vi "myRIO_BRig_RT__Case_Exp_State_initTrial_dispense.vi"(10 "input_state":T1, 11 "input_dataMTrig":u16[](array[numeric])) -> (0 "output_dispense__R":bool, 1 "output_dispense__L":bool, 2 "output_state":T1, 3 "output_dataMTrig":u16[](array[numeric]))   [LabVIEW 2014]
uses:
  myRIO_Gil_RT_v1__states.vi
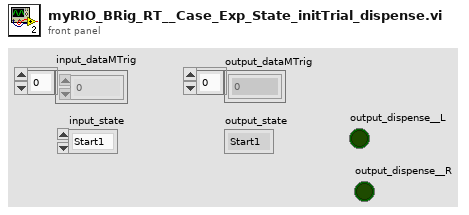
[diagram p1: front panel]
types:
  T1 = typedef "myRIO_Gil_RT_v1__states.vi" = enum16{"Start1", "Start2", "Start3", "initBlock", "initTrial", "initTrial_dispense_pre", "initTrial_dispense", "ENL1_pre", "ENL1", "ENL1Penalty_pre", "ENL1Penalty", "ENL2_pre", "ENL2", "ENL2Penalty_pre", "ENL2Penalty", "Cue1_pre", "Cue1", "Cue1Penalty_pre", "Cue1Penalty", "Cue2_pre", "Cue2", "Cue2Penalty_pre", "Cue2Penalty", "Selection_pre", "Selection", "SelectReward_pre", "SelectReward", "SelectRewardPost_pre", "SelectRewardPost", "SelectWrong_pre", "SelectWrong", "SelectTimeout_pre", "SelectTimeout", "SelectTimeout_post", "endTrial1", "endTrial2", "transferCheck", "transferPrepare", "transferCleanUp", "endBlock", "endExp"}
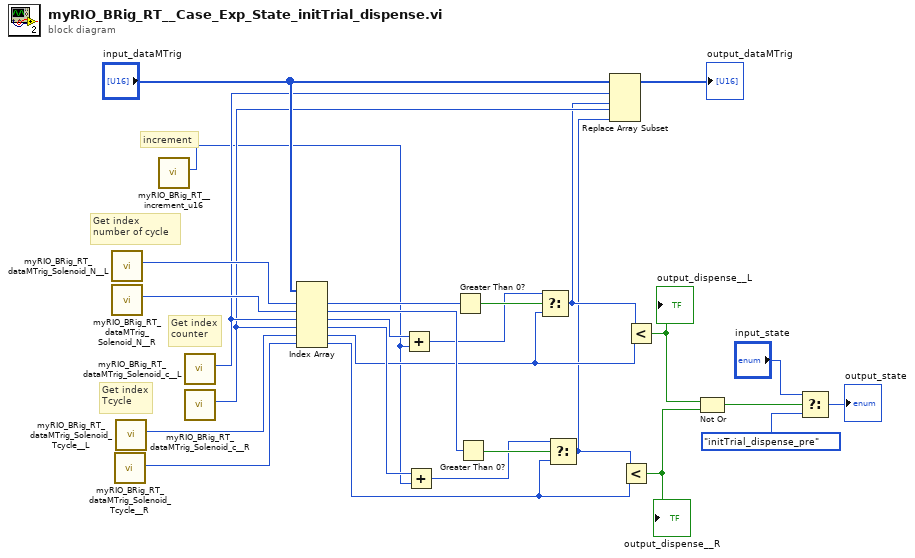
[diagram p0: block diagram]
diagram:
  # "increment"
  # "Get index\nTcycle"
  # "Get index\nnumber of cycle"
  # "Get index\ncounter"
  n1 = call "myRIO_BRig_RT_dataMTrig_Solenoid_N__L.vi"() -> ("output_Solenoid_N__L"=w27:i32)  [unwired: 11 in]
  n2 = call "myRIO_BRig_RT_dataMTrig_Solenoid_N__R.vi"() -> ("output_Solenoid_N__R"=w26:i32)  [unwired: 11 in]
  n3 = call "myRIO_BRig_RT_dataMTrig_Solenoid_Tcycle__R.vi"() -> ("output_Solenoid_Tcycle__R"=w24:i32)  [unwired: 11 in]
  n4 = call "myRIO_BRig_RT_dataMTrig_Solenoid_Tcycle__L.vi"() -> ("output_Solenoid_Tcycle__L"=w25:i32)  [unwired: 11 in]
  n5 = call "myRIO_BRig_RT__increment_u16.vi"() -> ("output_increment__u16"=w1:u16)  [unwired: 11 in]
  n6 = call "myRIO_BRig_RT_dataMTrig_Solenoid_c__L.vi"() -> ("output_Solenoid_c__L"=w11:i32)  [unwired: 11 in]
  n7 = call "myRIO_BRig_RT_dataMTrig_Solenoid_c__R.vi"() -> ("output_Solenoid_c__R"=w10:i32)  [unwired: 11 in]
  n8 = Index Array(array="input_dataMTrig", index #1=w27, index #2=w26, index #3=w11, index #4=w10, index #5=w25, index #6=w24) -> (element #1=w23:u16, element #2=w22:u16, element #3=w21:u16, element #4=w20:u16, element #5=w15:u16, element #6=w14:u16)
  n9 = Add(x=w21, y=w1) -> (x+y=w18:u16)
  n10 = Add(x=w20, y=w1) -> (x+y=w16:u16)
  n11 = Greater Than 0?(x=w23) -> (x > 0?=w19:bool)
  n12 = Greater Than 0?(x=w22) -> (x > 0?=w17:bool)
  n13 = Select(t=w18, s=w19, f=w15) -> (s? t:f=w9:u16)
  n14 = Select(t=w16, s=w17, f=w14) -> (s? t:f=w8:u16)
  n15 = Replace Array Subset(array="input_dataMTrig", new element #1=w9, index #1=w11, new element #2=w8, index #2=w10) -> (→"output_dataMTrig":u16[])
  n16 = Less?(x=w8, y=w14) -> (x < y?=w6:bool)
  "output_dispense__R" <- w6
  n17 = Less?(x=w9, y=w15) -> (x < y?=w7:bool)
  "output_dispense__L" <- w7
  n18 = Not Or(1:w6, 2:w7) -> (0:w5:bool)
  n19 = Select(t="input_state", s=w5, f=myRIO_Gil_RT_v1__states.vi."initTrial_dispense_pre") -> (s? t:f=→"output_state":T1)
